vi "Serial read all.vi"(8 "error in (no error)":errorcluster, 11 "VISA resource name":refnum<visa-resource-name>) -> (0 "error out":errorcluster, 1 "read strings":string[](array[string]), 3 "VISA resource name out":refnum<visa-resource-name>)   [LabVIEW 2017, in "Millennia V.lvclass"]
doc: "Reads all available strings from a given serial port. Useful after sending a string of commands, to read all the responses at once."
uses:
  Millennia V.lvclass
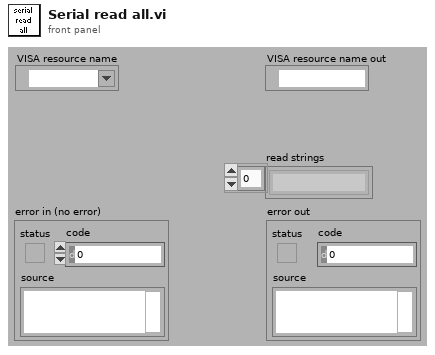
[diagram p1: front panel]
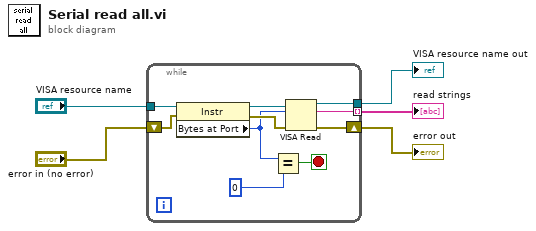
[diagram p0: block diagram]
diagram:
  n1 = while {
    tunnel: "VISA resource name" -> [w13]
    tunnel: [w12] -> w1
    tunnel: [w10] -> w5 mode=indexing
    shift-right: [w9] -> w2
    shift-left: "error in (no error)" -> [w8]
    stop <- w11 stop-if-true
    n2 = property class="Instr"(reference=w13, error in=w8) -> (reference out=w15:refnum<visa-resource-name>, error out=w14:errorcluster, "Bytes at Port"=w6:u32)
    n3 = Equal?(x=w6, y=0) -> (x = y?=w11:bool)
    n4 = VISA Read(VISA resource name=w15, byte count=w6, error in (no error)=w14) -> (VISA resource name out=w12:refnum<visa-resource-name>, read buffer=w10:string, error out=w9:errorcluster)  [unwired: 1 out]
  }
  "VISA resource name out" <- w1
  "read strings" <- w5
  "error out" <- w2
